vi "Dummy_process_loops.vi"   [LabVIEW 2017, in "labview-standard-library.lvlib" / "automode-scripting.lvlib"]
uses:
  automode-scripting.lvlib
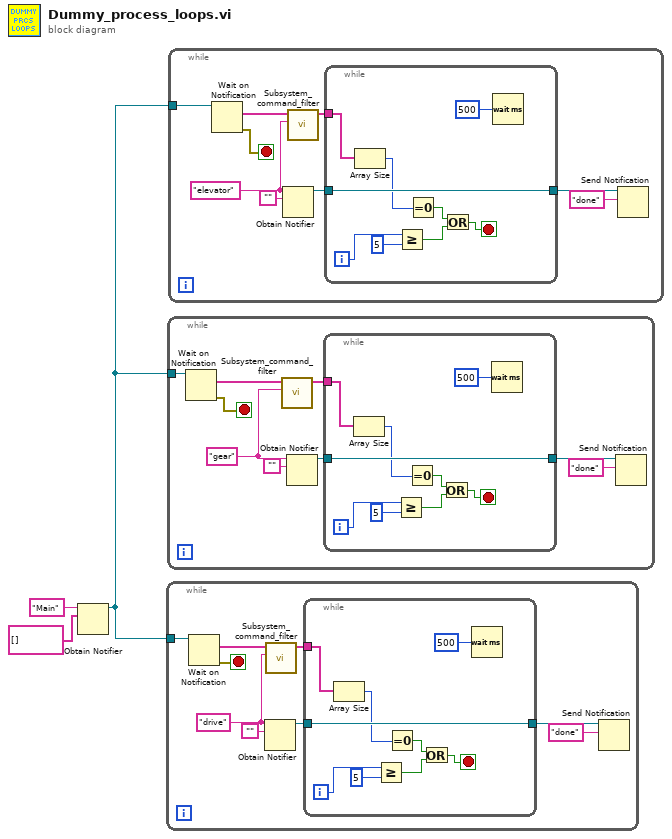
[diagram p0: block diagram]
diagram:
  n1 = Obtain Notifier(name (unnamed)="Main", notification data type=string[] [] ("appended array")) -> (notifier out=w3:refnum<notifier>)  [unwired: 2 in, 2 out]
  n2 = while {
    tunnel: w3 -> [w12]
    stop <- w4 stop-if-true
    w5 = "drive"
    n3 = Wait on Notification(notifier=w12) -> (notification=w11:string[], error out=w4:errorcluster)  [unwired: 3 in, 2 out]
    n4 = Obtain Notifier(name (unnamed)=w5, notification data type="") -> (notifier out=w6:refnum<notifier>)  [unwired: 2 in, 2 out]
    n5 = call "Subsystem_command_filter.vi"("Subsystem name"=w5, "Array of commands"=w11) -> ("Subsystem commands out"=w10:string[])  [unwired: 9 in]
    n6 = while {
      tunnel: w10 -> [w17]
      tunnel: w6 -> [w18]
      tunnel: [w18] -> w9
      i -> [w20]
      stop <- w15 stop-if-true
      n7 = Array Size(array=w17) -> (size(s)=w16:i32)
      n8 = Greater Or Equal?(x=w20, y=5) -> (x >= y?=w13:bool)
      n9 = Equal To 0?(x=w16) -> (x = 0?=w14:bool)
      n10 = Or(x=w14, y=w13) -> (x .or. y?=w15:bool)
      n11 = Wait (ms)(milliseconds to wait=u32 500) -> ()  [unwired: 1 out]
    }
    n12 = Send Notification(notification="done", notifier=w9) -> ()  [unwired: 1 in, 2 out]
  }
  n13 = while {
    tunnel: w3 -> [w30]
    stop <- w22 stop-if-true
    w23 = "gear"
    n14 = Wait on Notification(notifier=w30) -> (notification=w29:string[], error out=w22:errorcluster)  [unwired: 3 in, 2 out]
    n15 = call "Subsystem_command_filter.vi"("Subsystem name"=w23, "Array of commands"=w29) -> ("Subsystem commands out"=w28:string[])  [unwired: 9 in]
    n16 = Obtain Notifier(name (unnamed)=w23, notification data type="") -> (notifier out=w24:refnum<notifier>)  [unwired: 2 in, 2 out]
    n17 = while {
      tunnel: w28 -> [w35]
      tunnel: w24 -> [w36]
      tunnel: [w36] -> w27
      i -> [w38]
      stop <- w33 stop-if-true
      n18 = Array Size(array=w35) -> (size(s)=w34:i32)
      n19 = Greater Or Equal?(x=w38, y=5) -> (x >= y?=w31:bool)
      n20 = Equal To 0?(x=w34) -> (x = 0?=w32:bool)
      n21 = Or(x=w32, y=w31) -> (x .or. y?=w33:bool)
      n22 = Wait (ms)(milliseconds to wait=u32 500) -> ()  [unwired: 1 out]
    }
    n23 = Send Notification(notification="done", notifier=w27) -> ()  [unwired: 1 in, 2 out]
  }
  n24 = while {
    tunnel: w3 -> [w48]
    stop <- w40 stop-if-true
    w41 = "elevator"
    n25 = Wait on Notification(notifier=w48) -> (notification=w47:string[], error out=w40:errorcluster)  [unwired: 3 in, 2 out]
    n26 = Obtain Notifier(name (unnamed)=w41, notification data type="") -> (notifier out=w42:refnum<notifier>)  [unwired: 2 in, 2 out]
    n27 = call "Subsystem_command_filter.vi"("Subsystem name"=w41, "Array of commands"=w47) -> ("Subsystem commands out"=w46:string[])  [unwired: 9 in]
    n28 = while {
      tunnel: w46 -> [w53]
      tunnel: w42 -> [w54]
      tunnel: [w54] -> w45
      i -> [w56]
      stop <- w51 stop-if-true
      n29 = Array Size(array=w53) -> (size(s)=w52:i32)
      n30 = Greater Or Equal?(x=w56, y=5) -> (x >= y?=w49:bool)
      n31 = Equal To 0?(x=w52) -> (x = 0?=w50:bool)
      n32 = Or(x=w50, y=w49) -> (x .or. y?=w51:bool)
      n33 = Wait (ms)(milliseconds to wait=u32 500) -> ()  [unwired: 1 out]
    }
    n34 = Send Notification(notification="done", notifier=w45) -> ()  [unwired: 1 in, 2 out]
  }
